vi "Add Documentation to Interface Classes.vi"   [LabVIEW 2015]
doc: "<b> </b> <b> </b>\n©2016 Q Software Innovations, LLC (QSI)\nwritten by Quentin Alldredge\nproduced in LabVIEW 2015"
uses:
  Project Manipulation Scripts/Project Manipulation Scripts.lvlib
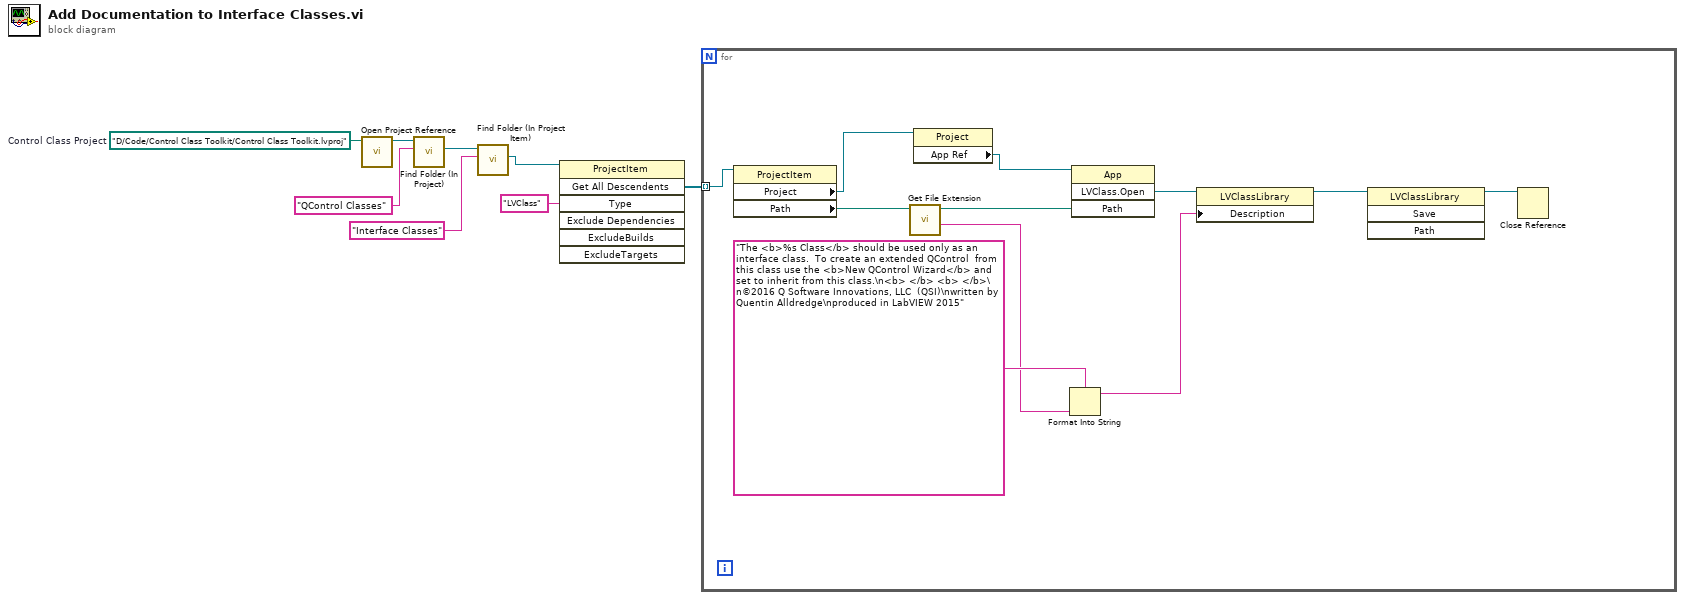
[diagram p0: block diagram]
diagram:
  w8 = path "D:/Code/Control Class Toolkit/Control Class Toolkit.lvproj"  # Control Class Project
  n1 = call "Open Project Reference.vi"("Project Path"=w8) -> ("Project out"=w7:refnum<vi>)  [unwired: 10 in]
  n2 = call "Find Folder (In Project).vi"("Folder Name"="QControl Classes", "Project in"=w7) -> ("Folder Refnum"=w3:refnum<vi>)  [unwired: 7 in, 2 out]
  n3 = call "Find Folder (In Project Item).vi"("Folder Name"="Interface Classes", "ProjectItem in"=w3) -> ("Folder Refnum"=w2:refnum<vi>)  [unwired: 7 in, 2 out]
  n4 = invoke class="ProjectItem" method="Get All Descendents"(reference=w2, "Type"="LVClass") -> ("All Descendents"=w4:refnum<vi>[])  [unwired: 5 in, 6 out]
  n5 = for {
    tunnel: w4 -> [w19] mode=indexing
    n6 = property class="ProjectItem"(reference=w19) -> ("Project"=w13:refnum<vi>, "Path"=w15:path)  [unwired: 1 in, 2 out]
    n7 = call <vilib>:"Get File Extension.vi"("file"=w15) -> ("filename without extension"=w14:string, "dup file"=w11:path)  [unwired: 6 in, 3 out]
    n8 = property class="Project"(reference=w13) -> ("App Ref"=w12:refnum<vi>)  [unwired: 1 in, 2 out]
    n9 = Format Into String(format string="The <b>%s Class</b> should be used only as an interface class.  To create an extended QControl  from this class use the <b>New QControl Wizard</b> and set to inherit from this class.\n<b> </b> <b> </b>\n©2016 Q Software Innovations, LLC  (QSI)\nwritten by Quentin Alldredge\nproduced in LabVIEW 2015" ("VI Description"), w14) -> (resulting string=w17:string)  [unwired: 2 in, 1 out]
    n10 = invoke class="App" method="LVClass.Open"(reference=w12, "Path"=w11) -> ("LVClass.Open"=w10:refnum<vi>)  [unwired: 2 in, 3 out]
    n11 = property class="LVClassLibrary"(reference=w10, "Description"=w17) -> (reference out=w18:refnum<vi>)  [unwired: 1 in, 1 out]
    n12 = invoke class="LVClassLibrary" method="Save"(reference=w18) -> (reference out=w9:refnum<vi>)  [unwired: 3 in, 3 out]
    n13 = Close Reference(reference=w9) -> ()  [unwired: 1 in, 1 out]
  }
